vi "Run Animations.vi"(8 "Error In":errorcluster, 10 "Frame Count":u64, 11 "Display Manager In":refnum<class "Display Manager.lvclass">) -> (0 "Error Out":errorcluster, 3 "Display Manager Out":refnum<class "Display Manager.lvclass">)   [LabVIEW 2021, in "Display Manager.lvclass"]
uses:
  Display Manager.lvclass
  Accessors/Display Elements/Get Display Elements.vi
  Accessors/Display Elements/Set Display Elements.vi
  Display Element/Display Element.lvclass
  Display Manager.lvclass/Display Manager.ctl
  Animation/Animation.lvclass
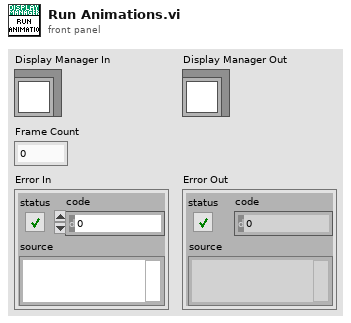
[diagram p1: front panel]
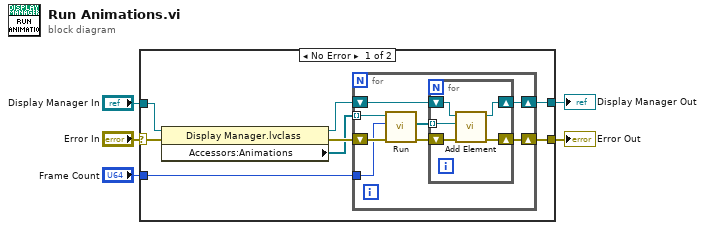
[diagram p0: block diagram]
diagram:
  n1 = case shown="No Error" "Error In" {
    selector: "Error In" -> [w12 w27]
    tunnel: "Display Manager In" -> [w13 w28]
    tunnel: [w7 w28] -> w3
    tunnel: [w9 w27] -> w2
    tunnel: "Frame Count" -> [w6 _]
    frame No Error {
      n2 = property class="Display Manager.lvclass"(reference=w13, error in=w12) -> (reference out=w8:refnum<class "Display Manager.lvclass">, error out=w11:errorcluster, "Accessors:Animations"=w10:refnum<class "Animation.lvclass">[])
      n3 = for {
        shift-right: [w15] -> w9
        shift-left: w11 -> [w20]
        tunnel: w10 -> [w21] mode=indexing
        shift-right: [w16] -> w7
        shift-left: w8 -> [w17]
        tunnel: w6 -> [w14]
        n4 = call-dynamic "Run.vi"("Error In"=w20, "Frame Count"=w14, "Animation In"=w21) -> ("Error Out"=w18:errorcluster, "Display Elements"=w19:refnum<class "Display Element.lvclass">[])  [unwired: 6 in, 1 out]
        n5 = for {
          tunnel: w19 -> [w24] mode=indexing
          shift-right: [w25] -> w15
          shift-left: w18 -> [w26]
          shift-right: [w22] -> w16
          shift-left: w17 -> [w23]
          n6 = call "Add Element.vi"("Error In"=w26, "New Element"=w24, "Display Manager In"=w23) -> ("Error Out"=w25:errorcluster, "Display Manager Out"=w22:refnum<class "Display Manager.lvclass">)  [unwired: 7 in]
        }
      }
    }
    frame Error {
    }
  }
  "Display Manager Out" <- w3
  "Error Out" <- w2
